vi "Pre Launch Init.vi"(11 "Vision in":refnum<class "Vision.lvclass">) -> (0 "error out":errorcluster, 3 "Vision out":refnum<class "Vision.lvclass">)   [LabVIEW 2021, in "Vision.lvlib" / "Vision.lvclass"]
doc: "(<B>Filename</B>: Actor Framework.lvlib:Actor.lvclass:Pre Launch Init.vi)\n\nDefines behavior that occurs after the Launch Nested Actor method is invoked but before the actor's Actor Core method begins running.\n\nBy default, this method does nothing. A descendant class may override it to define behavior."
uses:
  Vision.lvclass
  Vision.lvclass/Vision.ctl
  <vilib>/ActorFramework/Actor/Actor.lvclass
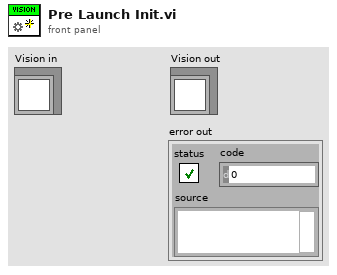
[diagram p1: front panel]
types:
  T1 = typedef "Image Type" = u32
  T2 = typedef "IMAQ Image.ctl" = refnum<image>
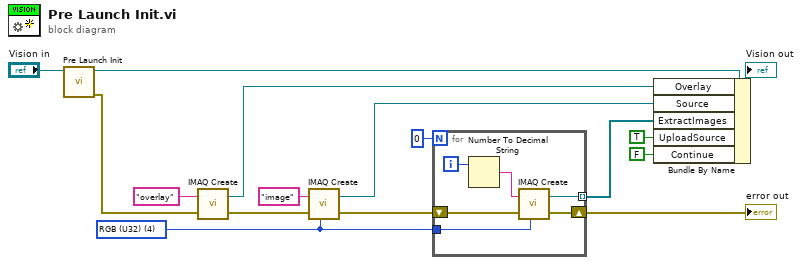
[diagram p0: block diagram]
diagram:
  w7 = T1 4 items=["Grayscale (U8)", "Grayscale (I16)", "Grayscale (SGL)", "Complex (CSG)", "RGB (U32)", "HSL (U32)", "RGB (U64)", "Grayscale (U16)"] ("Image Type")
  n1 = call-parent "Pre Launch Init.vi"("Actor in"="Vision in") -> ("error out"=w4:errorcluster, "Actor out"=w16:refnum<class "Vision.lvclass">)  [unwired: 9 in]
  n2 = call "IMAQ Create"("Image Name"="overlay", "error in (no error)"=w4) -> ("New Image"=w2:T2, "error out"=w3:errorcluster)  [unwired: 3 in]
  n3 = call "IMAQ Create"("Image Name"="image", "Image Type"=w7, "error in (no error)"=w3) -> ("New Image"=w12:T2, "error out"=w9:errorcluster)  [unwired: 2 in]
  n4 = for {
    N: 0 -> [_]
    tunnel: [w20] -> w11 mode=indexing
    shift-right: [w19] -> w10
    shift-left: w9 -> [w18]
    tunnel: w7 -> [w17]
    i -> [w22]
    n5 = Number To Decimal String(number=w22) -> (decimal integer string=w21:string)  [unwired: 1 in]
    n6 = call "IMAQ Create"("Image Name"=w21, "Image Type"=w17, "error in (no error)"=w18) -> ("New Image"=w20:T2, "error out"=w19:errorcluster)  [unwired: 2 in]
  }
  "error out" <- w10
  n7 = Bundle By Name(cluster=w16, "Overlay"=w2, "Source"=w12, "ExtractImages"=w11, "UploadSource"=TRUE, "Continue"=FALSE) -> (→"Vision out":refnum<class "Vision.lvclass">)
